vi "Create_File.vi"(1 "String":string="F:\\L0_Measurements_") -> (0 "path":path)   [LabVIEW 2012]
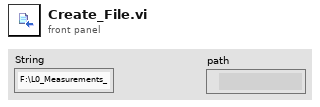
[diagram p1: front panel]
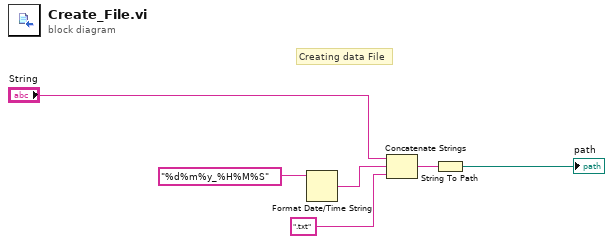
[diagram p0: block diagram]
diagram:
  # "Creating data File"
  n1 = Format Date/Time String(time format string (%c)="%d%m%y_%H%M%S") -> (date/time string=w6:string)  [unwired: 2 in]
  n2 = Concatenate Strings("String", w6, ".txt") -> (w3:string)
  n3 = String To Path(string=w3) -> (path=→"path":path)
